vi "SelectSettingsForUART.vi"() -> (1 "BaundRate":u32, 2 "COMPort":refnum<visa-resource-name>)   [LabVIEW 2014, in "Manipulator.lvclass"]
uses:
  Manipulator.lvclass
panel:
  in  "OK":bool
  in  "Ring":u32(ring)=9600 items=["115200"=115200, "57600"=57600, "38400"=38400, "19200"=19200, "9600"=9600, "4800"=4800]
  in  "VISA resource name":refnum<visa-resource-name>
  # "Select COM Port and Baund Rate then Confirm by OK button"
  # "COM PORT"
  # "BAUND RATE"
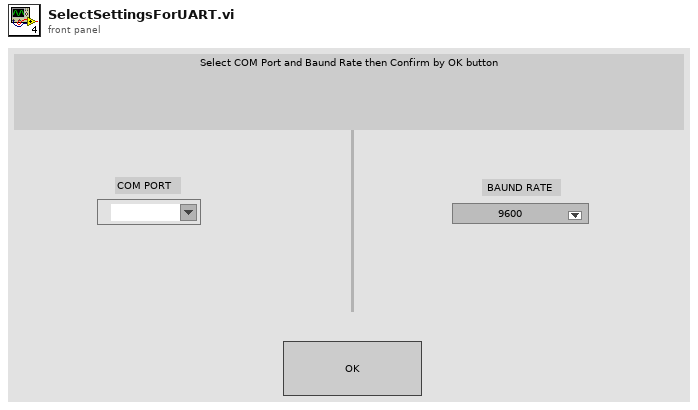
[diagram p1: front panel]
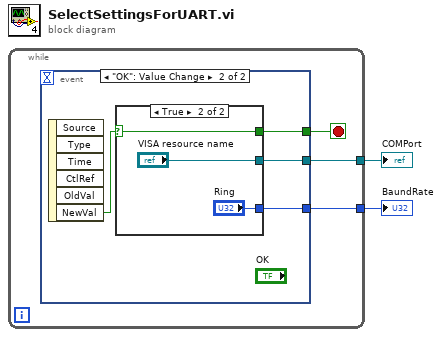
[diagram p0: block diagram]
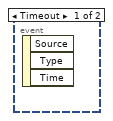
[diagram p2: hidden frame]
diagram:
  n1 = while {
    tunnel: [w4] -> w2
    tunnel: [w3] -> w1
    stop <- w5 stop-if-true
    n2 = event shown="[1] \"OK\": Value Change" {
      selector: _ -> [_ _]
      dyn-events: _ -> [_ _]
      timeout: _ -> [_ _]
      tunnel: [_ w8] -> w5
      tunnel: [_ w7] -> w4
      tunnel: [_ w6] -> w3
      event Timeout {
        n3 = event-data() -> ()  [unwired: 1 in, 3 out]
      }
      event "OK": Value Change {
        n4 = event-data() -> ("NewVal"=w9:bool)  [unwired: 1 in, 5 out]
        n5 = case shown="True" w9 {
          selector: w9 -> [_ w12]
          tunnel: [_ w12] -> w8
          tunnel: [_ "VISA resource name"] -> w7
          tunnel: [_ "Ring"] -> w6
          frame False {
          }
          frame True {
          }
        }
      }
    }
  }
  "COMPort" <- w2
  "BaundRate" <- w1
